vi "GetPlayerText.vi"(3 "Player":T1) -> (1 "Text":string)   [LabVIEW 2020]
uses:
  controls/Player.ctl
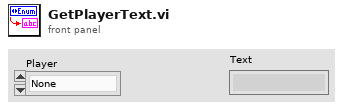
[diagram p1: front panel]
types:
  T1 = typedef "Player.ctl" = enum16{"None", "Player 1", "Player 2"}
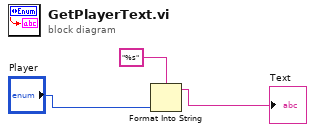
[diagram p0: block diagram]
diagram:
  n1 = Format Into String(format string="%s", "Player") -> (resulting string=→"Text":string)  [unwired: 2 in, 1 out]
